vi "Read Action sequence.vi"(8 "error in (no error)":errorcluster, 11 "Sequence in":refnum<class "Action-sequence.lvclass">) -> (0 "error out":errorcluster, 2 "Action sequence":refnum<class "Action.lvclass">[](array[class]), 3 "Sequence out":refnum<class "Action-sequence.lvclass">)   [LabVIEW 2013, in "PowderDeposition.lvlib" / "Action-sequence.lvclass"]
uses:
  Action-sequence.lvclass
  Action/Action.lvclass
  Action-sequence.lvclass/Action-sequence.ctl
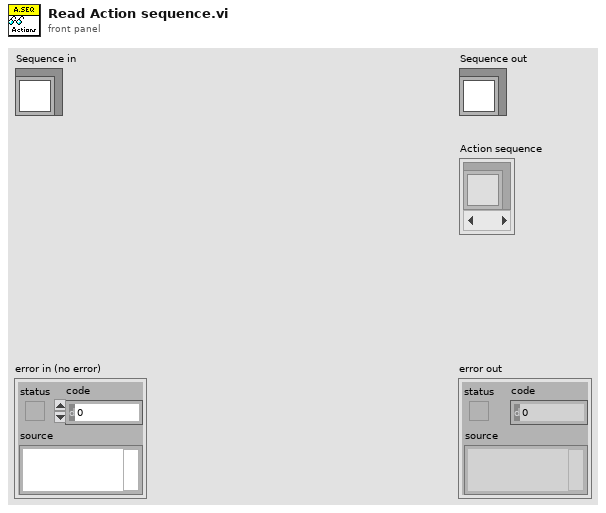
[diagram p1: front panel]
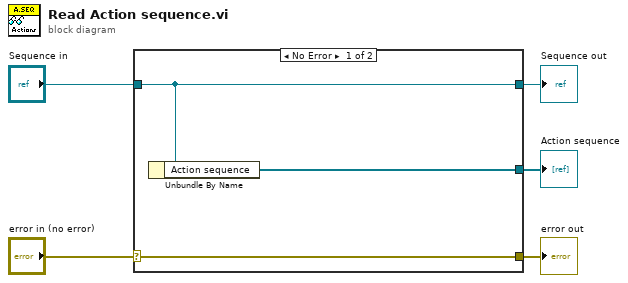
[diagram p0: block diagram]
diagram:
  n1 = case shown="No Error" "error in (no error)" {
    selector: "error in (no error)" -> [w8 w9]
    tunnel: [w8 w9] -> w4
    tunnel: [w7 w10] -> w2
    tunnel: "Sequence in" -> [w7 w10]
    tunnel: [w6 _] -> w1
    frame No Error {
      n2 = Unbundle By Name(w7) -> ("Action sequence"=w6:refnum<class "Action.lvclass">[])
    }
    frame Error {
    }
  }
  "error out" <- w4
  "Sequence out" <- w2
  "Action sequence" <- w1
